vi "GetCharacteristics.vi"(8 "error in":errorcluster, 11 "Measure in":refnum<class "Measure.lvclass">) -> (0 "error out":errorcluster, 2 "Characteristics":refnum<class "Characteristic.lvclass">[](array[class]), 3 "Measure out":refnum<class "Measure.lvclass">)   [LabVIEW 2021, in "ProligentXMLGenerator.lvlib" / "Measure.lvclass"]
doc: "Defines a comment associated to the measure."
uses:
  Measure.lvclass
  Measure.lvclass/Measure.ctl
  Model/Characteristic/Characteristic.lvclass
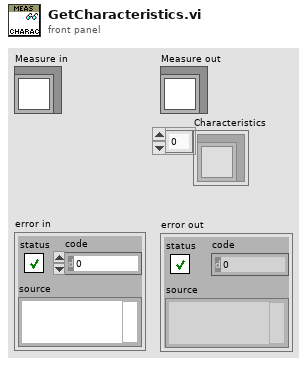
[diagram p1: front panel]
types:
  T1 = typedef "ProligentXMLGenerator.lvlib/Measure.lvclass/Data.ctl" = cluster{"Name":string, "Type":refnum<class "MeasureKind.lvclass">, "Precision":refnum<class "UnsignedByte.lvclass">, "Limit":refnum<class "MeasureLimit.lvclass">, "Characteristics":refnum<class "Characteristic.lvclass">[], "FailureReferences":refnum<class "FailureReference.lvclass">[], "CustomData":refnum<class "CustomData.lvclass">, "MeasureId":refnum<class "Guid.lvclass">, "MeasureTime":refnum<class "DateTime.lvclass">, "Comments":refnum<class "NonNullableString_TruncateAt_255.lvclass">, "Unit":refnum<class "NonEmptyString_30.lvclass">, "Symbol":refnum<class "NonEmptyString_20.lvclass">, "MeasureExecutionStatus":refnum<class "ExecutionStatus.lvclass">}
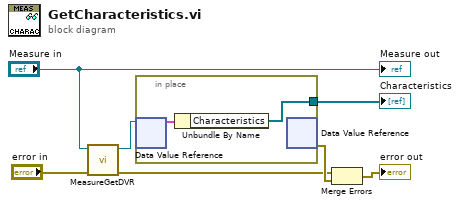
[diagram p0: block diagram]
diagram:
  n1 = call "MeasureGetDVR.vi"("error in"="error in", "Measure"="Measure in") -> ("error out"=w1:errorcluster, "DVRReference"=w6:refnum<data-value>)  [unwired: 8 in]
  n2 = in-place "In Place Element Structure" {
    in-place-border: [w8] -> w2
    n3 = in-place-dvr #1(w6) -> (w9:T1)  [unwired: 1 out]
    n4 = Unbundle By Name(w9) -> ("Characteristics"=w8:refnum<class "Characteristic.lvclass">[])
    n5 = in-place-dvr #1() -> (w7:errorcluster)  [unwired: 1 in, 1 out]
  }
  "Characteristics" <- w2
  n6 = Merge Errors(w1, w7) -> (→"error out":errorcluster)
  "Measure out" <- "Measure in"
